vi "Read EEPROM Addresses.vi"(8 "error in (no error)":errorcluster, 10 "Addresses":u16[](array[numeric]), 11 "Refnum in":refnum<k20>) -> (0 "error out":errorcluster, 2 "Data":u8[](array[numeric]), 3 "Refnum out":refnum<k20>)   [LabVIEW 2016, in "SMI.lvlib" / "C Series Module.lvclass"]
uses:
  C Series Module.lvclass
  <vilib>/Utility/error.llb/Error Cluster From Error Code.vi
  <vilib>/rvi/errors/niLvFpgaAdjustHostInterfaceError.vi
  <vilib>/rvi/interface/nirviReadWriteControl/nirviReadWriteControl.xnode
  NiFpgaLv.dll
  <vilib>/rvi/interface/Simulation/niFpgaSimulationCallBeginRW.vi
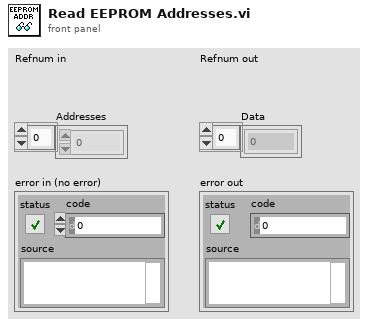
[diagram p1: front panel]
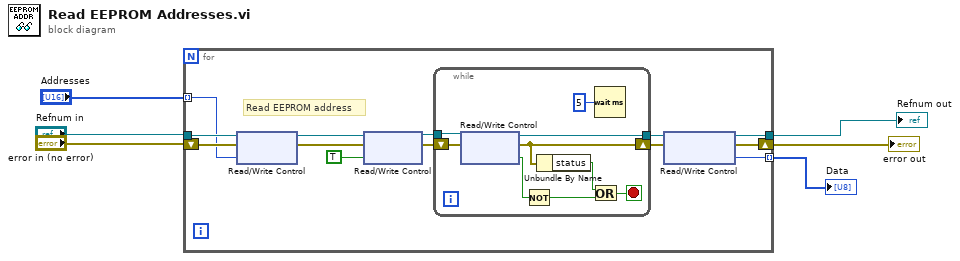
[diagram p0: block diagram]
diagram:
  n1 = for {
    shift-right: [w9] -> w1
    shift-left: "error in (no error)" -> [w19]
    tunnel: "Refnum in" -> [w18]
    tunnel: [w12] -> w2
    tunnel: "Addresses" -> [w8] mode=indexing
    tunnel: [w7] -> w6 mode=indexing
    # "Read EEPROM address"
    n2 = xnode "Read/Write Control"("FPGA VI Reference In"=w18, "error in"=w19, "Address"=w8) -> ("FPGA VI Reference Out"=w16:refnum<k20>, "error out"=w15:errorcluster)
    n3 = xnode "Read/Write Control"("FPGA VI Reference In"=w16, "error in"=w15, "Execute"=TRUE) -> ("FPGA VI Reference Out"=w17:refnum<k20>, "error out"=w14:errorcluster)
    n4 = while {
      shift-right: [w25] -> w10
      shift-left: w14 -> [w28]
      tunnel: w17 -> [w27]
      tunnel: [w26] -> w11
      stop <- w21 stop-if-true
      n5 = xnode "Read/Write Control"("FPGA VI Reference In"=w27, "error in"=w28) -> ("FPGA VI Reference Out"=w26:refnum<k20>, "error out"=w25:errorcluster, "Execute"=w24:bool)
      n6 = Not(x=w24) -> (.not. x?=w22:bool)
      n7 = Unbundle By Name(w25) -> ("status"=w23:bool)
      n8 = Or(x=w23, y=w22) -> (x .or. y?=w21:bool)
      n9 = Wait (ms)(milliseconds to wait=u32 5) -> ()  [unwired: 1 out]
    }
    n10 = xnode "Read/Write Control"("FPGA VI Reference In"=w11, "error in"=w10) -> ("FPGA VI Reference Out"=w12:refnum<k20>, "error out"=w9:errorcluster, "Data Read"=w7:u8)
  }
  "Data" <- w6
  "Refnum out" <- w2
  "error out" <- w1
